vi "Ej 16 Histeresis.vi"() -> ()   [LabVIEW 2021]
panel:
  in  "Temperatura":dbl
  out "Actuador":bool
  in  "?":bool
  # "Histeresis"
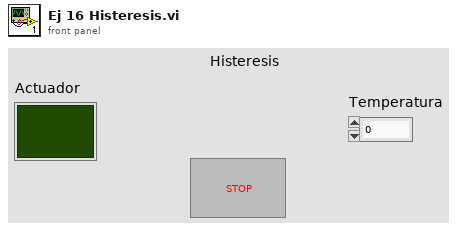
[diagram p1: front panel]
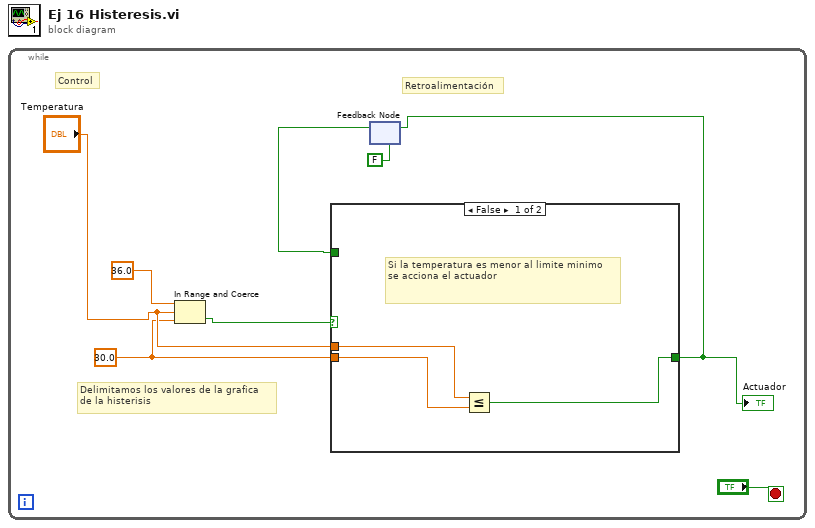
[diagram p0: block diagram]
diagram:
  n1 = while {
    stop <- "?" stop-if-true
    w5 = 30.0 ("lower limit")
    # "Control"
    # "Retroalimentación"
    # "Delimitamos los valores de la grafica \nde la histerisis"
    n2 = In Range and Coerce(upper limit=36.0, x="Temperatura", lower limit=w5) -> (In Range?=w7:bool)  [unwired: 1 out]
    n3 = feedback #1(FALSE) -> (w2:bool)
    n4 = case shown="False" w7 {
      tunnel: "Temperatura" -> [w11 _]
      tunnel: w5 -> [w10 _]
      tunnel: [w9 w12] -> w4
      tunnel: w2 -> [_ w12]
      frame False {
        # "Si la temperatura es menor al limite minimo\nse acciona el actuador"
        n5 = Less Or Equal?(x=w11, y=w10) -> (x <= y?=w9:bool)
      }
      frame True {
        # "Si la condicion es verdadera \nno se acciona el actuador"
      }
    }
    "Actuador" <- w4
    n6 = feedback-in #1(w4) -> ()
  }
